vi "Write Event Type.vi"(8 "error in (no error)":errorcluster, 10 "Event Type":T1(ring), 11 "PulseData in":refnum<class "PulseData.lvclass">) -> (0 "error out":errorcluster, 3 "PulseData out":refnum<class "PulseData.lvclass">)   [LabVIEW 2013, in "Controls Log Monitor.lvlib" / "PulseData.lvclass"]
uses:
  PulseData.lvclass
  PulseData.lvclass/PulseData.ctl
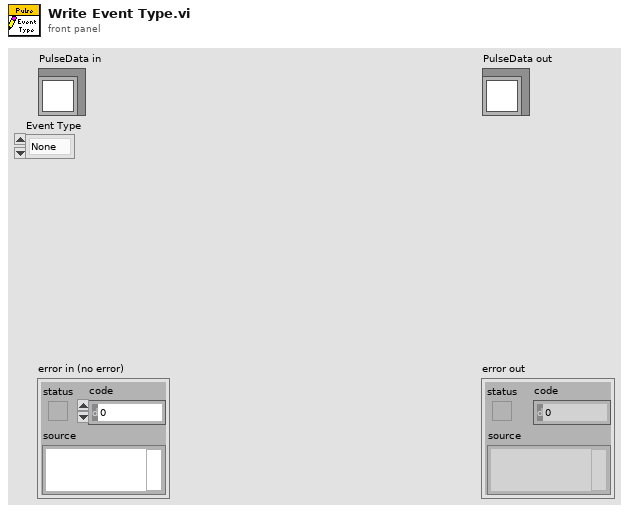
[diagram p1: front panel]
types:
  T1 = enum16{"None", "Tune", "Periodic Capture", "Spark Trigger"}
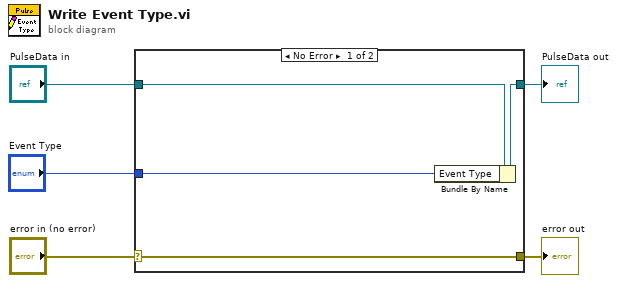
[diagram p0: block diagram]
diagram:
  n1 = case shown="No Error" "error in (no error)" {
    selector: "error in (no error)" -> [w9 w10]
    tunnel: [w9 w10] -> w4
    tunnel: [w8 w11] -> w2
    tunnel: "PulseData in" -> [w6 w11]
    tunnel: "Event Type" -> [w7 _]
    frame No Error {
      n2 = Bundle By Name(cluster=w6, "Event Type"=w7) -> (w8:refnum<class "PulseData.lvclass">)
    }
    frame Error {
    }
  }
  "error out" <- w4
  "PulseData out" <- w2
